vi "StartCAN.vi"() -> ()   [LabVIEW 2018]
uses:
  <vilib>/xnet/xnet.llb/XNET Frame CAN.ctl
  <vilib>/xnet/xnet.llb/XNET Frame Type CAN.ctl
  <vilib>/xnet/xnet.llb/XNET CAN Comm State.ctl
  <vilib>/xnet/xnet.llb/XNET Control Scope.ctl
  <vilib>/xnet/xnet.llb/XNET Create Session (Frame Input Queued).vi
  <vilib>/xnet/xnet.llb/XNET Create Session (Signal Output Single-point).vi
  <vilib>/xnet/xnet.llb/XNET Write (Frame CAN).vi
  <vilib>/xnet/xnet.llb/XNET Read (State CAN Comm).vi
  <vilib>/xnet/xnet.llb/XNET Wait (Interface Communicating).vi
  <resource>/objmgr/xnet.rc
panel:
  out "DSC Write Session out":refnum<k21>
  out "Read Session out":refnum<k21>
  out "Tester Write Session out":refnum<k21>
  out "Protocol":u32(ring) items=["CAN"=0, "FlexRay"=1, "LIN"=2, "Ethernet"=3, "Unknown"=4294967294]
  out "CAN:Transceiver Capability":u32(ring) items=["HS"=0, "LS"=1, "XS"=3, "XS (HS/LS)"=4]
  out "CAN:Termination Capability":u32(ring) items=["No", "Yes"]
  in  "CAN Interface":refnum<k21>
  out "CAN:I/O Mode":u32(ring) items=["CAN 2.0", "CAN FD", "CAN FD+BRS"]
  in  "64bit Baud Rate":u64
  out "XNET Database":refnum<k21>
  out "CAN DB":string
  in  "CAN Database":string
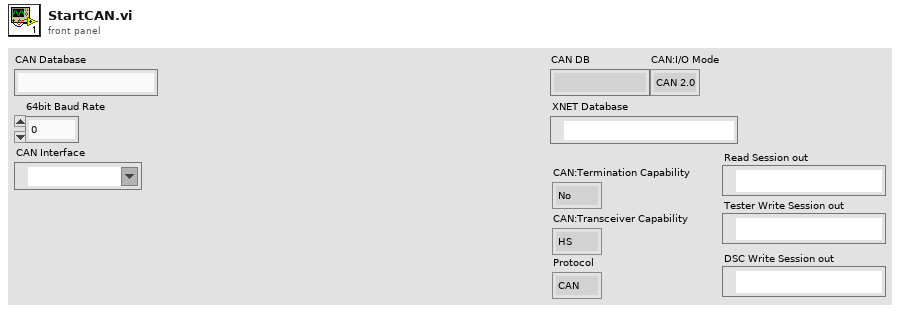
[diagram p1: front panel]
types:
  T1 = typedef "XNET Frame CAN.ctl" = cluster{"timestamp":timestamp, "payload":u8[], "identifier":u32, "type":T2, "extended?":bool, "echo?":bool}
  T2 = typedef "XNET Frame Type CAN.ctl" = u8
  T3 = cluster{"Comment":string, "Default Payload":u8[], "Identifier":u32, "Name (Short)":string, "Payload Length":u32, "PDU_Mapping":cluster{"PDU":string, "Start Bit":u32, "Update Bit":i32}[], "CAN:Extended Identifier?":bool, "CAN:Timing Type":u32, "CAN:Transmit Time":dbl, "CAN:I/O Mode":u32}
  T4 = cluster{"Comment":string, "Default Payload":u8[], "Identifier":u32, "Name (Short)":string, "Payload Length":u32, "PDU_Mapping":cluster{"PDU":string, "Start Bit":u32, "Update Bit":i32}[], "CAN:Extended Identifier?":bool, "CAN:Timing Type":u32, "CAN:Transmit Time":dbl, "CAN:I/O Mode":u32}[]
  T5 = typedef "XNET CAN Comm State.ctl" = u8
  T6 = typedef "XNET CAN Comm.ctl" = cluster{"fault code":i32, "fault?":bool, "communication state":T5, "last error":T7, "receive error counter":u8, "transmit error counter":u8, "transceiver error?":bool, "sleep?":bool}
  T7 = typedef "XNET CAN Last Err.ctl" = u8
  T8 = typedef "XNET Control Scope.ctl" = u32
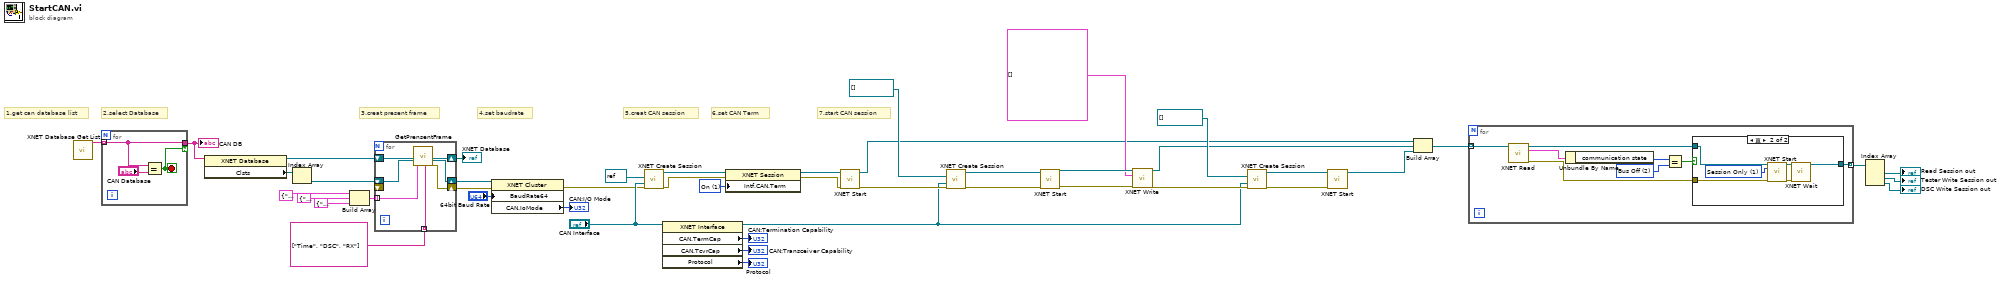
[diagram p0: block diagram]
diagram:
  w23 = u32 1 items=["Off", "On"] ("Interface:CAN:Termination")
  # "6.set CAN Term"
  # "7.start CAN session"
  # "5.creat CAN session"
  # "4.set baudrate"
  # "3.creat present frame"
  # "2.select Database"
  # "1.get can database list"
  n1 = call <vilib>:"XNET Database Get List.vi"() -> ("array of alias"=w46:string[])  [unwired: 13 in, 2 out]
  n2 = for {
    tunnel: w46 -> [w48] mode=indexing
    tunnel: [w48] -> w45 if=w47
    stop <- w47 stop-if-true
    n3 = Equal?(x=w48, y="CAN Database") -> (x = y?=w47:bool)
  }
  "CAN DB" <- w45
  n4 = property class="XNET Database"(reference=w45) -> (reference out=w43:refnum<k21>, "Clsts"=w44:refnum<k21>[])  [unwired: 1 in, 1 out]
  n5 = Index Array(array=w44) -> (element=w42:refnum<k21>)  [unwired: 1 in]
  n6 = Build Array(T3 {"Comment"="DSC", "Default Payload"=[0, 0, 0, 0, 0, 0, 0, 0], "Identifier"=1714, "Name (Short)"="Time", "Payload Length"=8, "PDU_Mapping"=[], "CAN:Extended Identifier?"=FALSE, "CAN:Timing Type"=0, "CAN:Transmit Time"=0.001, "CAN:I/O Mode"=0} ("New Frame Properties"), T3 {"Comment"="DSC", "Default Payload"=[0, 0, 0, 0, 0, 0, 0, 0], "Identifier"=402391172, "Name (Short)"="DSC", "Payload Length"=8, "PDU_Mapping"=[], "CAN:Extended Identifier?"=TRUE, "CAN:Timing Type"=1, "CAN:Transmit Time"=0.001, "CAN:I/O Mode"=0} ("New Frame Properties"), T3 {"Comment"="RX", "Default Payload"=[0, 127, 0, 0, 0, 0, 0, 0], "Identifier"=402522244, "Name (Short)"="RX", "Payload Length"=8, "PDU_Mapping"=[], "CAN:Extended Identifier?"=TRUE, "CAN:Timing Type"=1, "CAN:Transmit Time"=0.001, "CAN:I/O Mode"=0} ("New Frame Properties")) -> (w37:T4)
  n7 = for {
    shift-right: [w54] -> w36
    shift-left: w43 -> [w56]
    shift-right: [w53] -> w35
    shift-left: w42 -> [w55]
    tunnel: string[] ["Time", "DSC", "RX"] -> [w52] mode=indexing
    tunnel: w37 -> [w51] mode=indexing
    shift-right: [w50] -> w32
    shift-left: _ -> [_]
    n8 = call "GetPrensentFrame.vi"("database in"=w56, "Cluster::"=w55, "New Frame Properties"=w51, "frame name"=w52) -> ("database out"=w54:refnum<k21>, "target cluster out"=w53:refnum<k21>, "error out"=w50:errorcluster)  [unwired: 21 in]
  }
  "XNET Database" <- w36
  n9 = property class="XNET Cluster"(reference=w35, error in=w32, "BaudRate64"="64bit Baud Rate") -> (error out=w26:errorcluster, "CAN.IoMode"=→"CAN:I/O Mode":u32)  [unwired: 1 out]
  n10 = call-poly <vilib>:"XNET Create Session.vi"("frame"=refnum<k21> refnum, "interface"="CAN Interface", "error in (no error)"=w26) -> ("session out"=w25:refnum<k21>, "error out"=w24:errorcluster)  [unwired: 11 in]
  n11 = property class="XNET Interface"(reference="CAN Interface") -> (reference out=w11:refnum<k21>, "CAN.TermCap"=→"CAN:Termination Capability":u32, "CAN.TcvrCap"=→"CAN:Transceiver Capability":u32, "Protocol"=→"Protocol":u32)  [unwired: 1 in, 1 out]
  n12 = property class="XNET Session"(reference=w25, error in=w24, "Intf.CAN.Term"=w23) -> (reference out=w22:refnum<k21>, error out=w21:errorcluster)
  n13 = call <vilib>:"XNET Start.vi"("session in"=w22, "error in (no error)"=w21) -> ("session out"=w8:refnum<k21>, "error out"=w19:errorcluster)  [unwired: 12 in]
  n14 = call-poly <vilib>:"XNET Create Session.vi"("signal list"=refnum<k21>[] [], "interface"=w11, "error in (no error)"=w19) -> ("session out"=w18:refnum<k21>, "error out"=w17:errorcluster)  [unwired: 11 in]
  n15 = call <vilib>:"XNET Start.vi"("session in"=w18, "error in (no error)"=w17) -> ("session out"=w16:refnum<k21>, "error out"=w15:errorcluster)  [unwired: 12 in]
  n16 = call-poly <vilib>:"XNET Write.vi"("session in"=w16, "data"=T1[] [], "error in (no error)"=w15) -> ("session out"=w7:refnum<k21>, "error out"=w12:errorcluster)  [unwired: 11 in]
  n17 = call-poly <vilib>:"XNET Create Session.vi"("signal list"=refnum<k21>[] [], "interface"=w11, "error in (no error)"=w12) -> ("session out"=w10:refnum<k21>, "error out"=w9:errorcluster)  [unwired: 11 in]
  n18 = call <vilib>:"XNET Start.vi"("session in"=w10, "error in (no error)"=w9) -> ("session out"=w6:refnum<k21>)  [unwired: 12 in, 1 out]
  n19 = Build Array(w8, w7, w6) -> (w5:refnum<k21>[])
  n20 = for {
    tunnel: w5 -> [w64] mode=indexing
    tunnel: [w57] -> w4 mode=indexing
    w61 = T5 2 items=["Error Active", "Error Passive", "Bus Off", "Init"] ("y")
    n21 = call-poly <vilib>:"XNET Read.vi"("session in"=w64) -> ("session out"=w59:refnum<k21>, "CAN comm"=w63:T6, "error out"=w58:errorcluster)  [unwired: 12 in]
    n22 = Unbundle By Name(w63) -> ("communication state"=w62:T5)
    n23 = Equal?(x=w62, y=w61) -> (x = y?=w60:bool)
    n24 = case shown="真" w60 {
      tunnel: w59 -> [w65 w71]
      tunnel: w58 -> [_ w69]
      tunnel: [w65 w66] -> w57
      frame False {
      }
      frame True {
        w67 = T8 1 items=["Normal", "Session Only", "Interface Only", "Session Only Blocking"] ("scope (normal)")
        n25 = call <vilib>:"XNET Start.vi"("session in"=w71, "scope (normal)"=w67, "error in (no error)"=w69) -> ("session out"=w70:refnum<k21>, "error out"=w68:errorcluster)  [unwired: 11 in]
        n26 = call-poly <vilib>:"XNET Wait.vi"("session in"=w70, "error in (no error)"=w68) -> ("session out"=w66:refnum<k21>)  [unwired: 12 in, 1 out]
      }
    }
  }
  n27 = Index Array(array=w4) -> (element #1=→"Read Session out":refnum<k21>, element #2=→"Tester Write Session out":refnum<k21>, element #3=→"DSC Write Session out":refnum<k21>)  [unwired: 3 in]
